vi "Convert Mass to DAC.vi"(0 "Mass":dbl, 1 "Calibration Table":dbl[][](array[numeric]) format="%.2f") -> (2 "DAC Value":dbl, 3 "Slope":dbl, 4 "UpperIndex":i32, 5 "LowerIndex":i32)   [LabVIEW 2018]
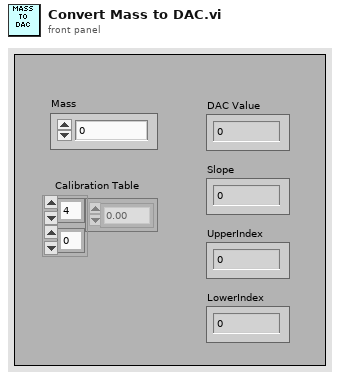
[diagram p1: front panel]
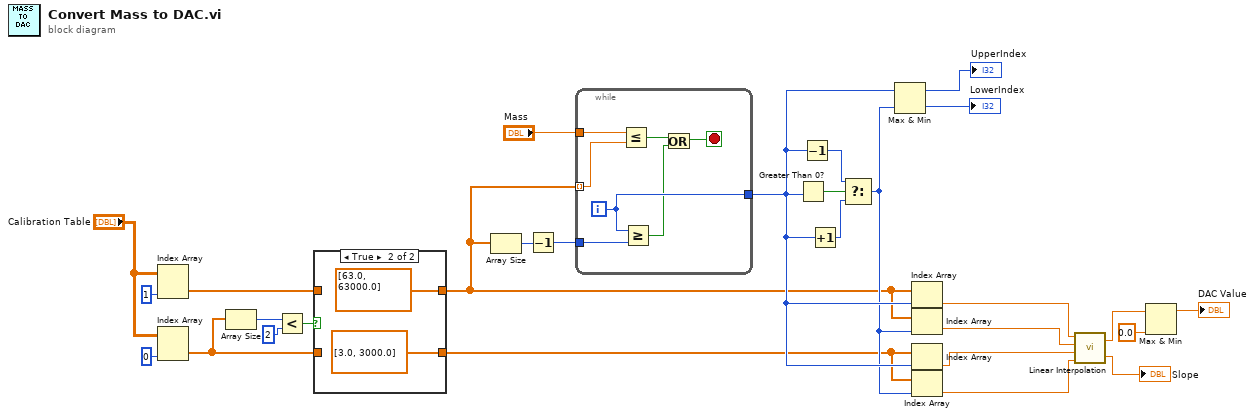
[diagram p0: block diagram]
diagram:
  n1 = Index Array(array="Calibration Table", index (col)=1 ("Index")) -> (element=w22:dbl[])  [unwired: 1 in]
  n2 = Index Array(array="Calibration Table", index (col)=0 ("Index")) -> (element=w23:dbl[])  [unwired: 1 in]
  n3 = Array Size(array=w23) -> (size(s)=w26:i32)
  n4 = Less?(x=w26, y=2) -> (x < y?=w24:bool)
  n5 = case shown="True" w24 {
    tunnel: w23 -> [w29 _]
    tunnel: w22 -> [w30 _]
    tunnel: [w29 dbl[] [3.0, 3000.0]] -> w9
    tunnel: [w30 dbl[] [63.0, 63000.0]] -> w10
    frame False {
    }
    frame True {
    }
  }
  n6 = Array Size(array=w10) -> (size(s)=w19:i32)
  n7 = Decrement(x=w19) -> (x-1=w18:i32)
  n8 = while {
    tunnel: w10 -> [w39] mode=indexing
    tunnel: "Mass" -> [w38]
    tunnel: [w37] -> w12
    tunnel: w18 -> [w33]
    i -> [w37]
    stop <- w36 stop-if-true
    n9 = Less Or Equal?(x=w38, y=w39) -> (x <= y?=w35:bool)
    n10 = Greater Or Equal?(x=w37, y=w33) -> (x >= y?=w34:bool)
    n11 = Or(x=w35, y=w34) -> (x .or. y?=w36:bool)
  }
  n12 = Greater Than 0?(x=w12) -> (x > 0?=w17:bool)
  n13 = Decrement(x=w12) -> (x-1=w16:i32)
  n14 = Increment(x=w12) -> (x+1=w15:i32)
  n15 = Select(t=w16, s=w17, f=w15) -> (s? t:f=w11:i32)
  n16 = Max & Min(x=w12, y=w11) -> (max(x,y)=→"UpperIndex":i32, min(x,y)=→"LowerIndex":i32)
  n17 = Index Array(array=w10, index=w12) -> (element=w8:dbl)
  n18 = Index Array(array=w10, index=w11) -> (element=w7:dbl)
  n19 = Index Array(array=w9, index=w12) -> (element=w6:dbl)
  n20 = Index Array(array=w9, index=w11) -> (element=w5:dbl)
  n21 = call "Linear Interpolation.vi"("X1"=w8, "X2"=w7, "Y1"=w6, "Y2"=w5) -> ("Y"=w3:dbl, "Slope"=→"Slope":dbl)  [unwired: 1 in]
  n22 = Max & Min(x=w3, y=0.0) -> (max(x,y)=→"DAC Value":dbl)  [unwired: 1 out]
